vi "Disconnect.vi"(8 "error in (no error)":errorcluster, 11 "connection ID":i32=-1) -> (0 "error out":errorcluster)   [LabVIEW 2009, in "MicroDAQ.lvlib"]
doc: "Disconnects device."
uses:
  <instrlib>/MicroDAQ/MicroDAQ.lvlib
  <instrlib>/MicroDAQ/Mlink library wraper/mlink.lvlib
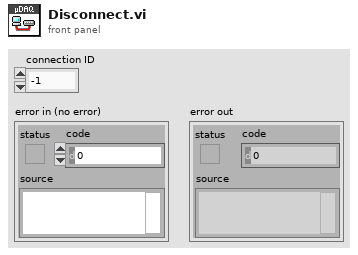
[diagram p1: front panel]
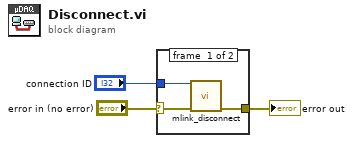
[diagram p0: block diagram]
diagram:
  n1 = case shown="No Error" "error in (no error)" {
    selector: "error in (no error)" -> [w6 w7]
    tunnel: "connection ID" -> [w5 _]
    tunnel: [w4 w7] -> w1
    frame #0 {
      n2 = call <instrlib>:"mlink_disconnect.vi"("error in (no error)"=w6, "connection ID"=w5) -> ("error out"=w4:errorcluster)  [unwired: 9 in]
    }
    frame #1 {
    }
  }
  "error out" <- w1
